vi "uTTA_SetDUT_Name.vi"(8 "error in":errorcluster, 10 "DUT Name":string, 11 "VISA Refnum in":refnum<visa-resource-name>) -> (0 "error out":errorcluster, 2 "Received":string, 3 "VISA Refnum out":refnum<visa-resource-name>)   [LabVIEW 2021]
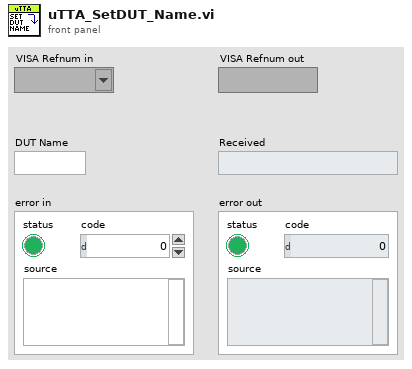
[diagram p1: front panel]
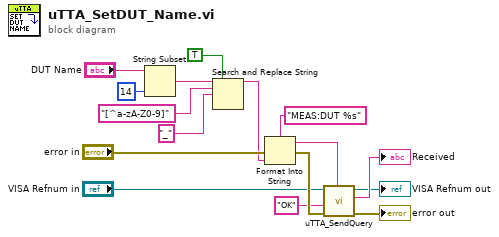
[diagram p0: block diagram]
diagram:
  n1 = String Subset(string="DUT Name", length (rest)=14 ("length (rest)")) -> (substring=w3:string)  [unwired: 1 in]
  n2 = Search and Replace String(replace all?=TRUE ("replace all? (F)"), input string=w3, search string="[^a-zA-Z0-9]", replace string="_" ("replace string (\"\")")) -> (result string=w2:string)  [unwired: 4 in, 3 out]
  n3 = Format Into String(format string="MEAS:DUT %s", error in="error in", w2) -> (resulting string=w13:string, error out=w15:errorcluster)  [unwired: 1 in]
  n4 = call "uTTA_SendQuery.vi"("Send String"=w13, "error in (no error)"=w15, "Response Qualifier(\"\")"="OK" ("Response Qualifier(\"\")"), "VISA Refnum in"="VISA Refnum in") -> ("error out"=→"error out":errorcluster, "Received"=→"Received":string, "VISA Refnum out"=→"VISA Refnum out":refnum<visa-resource-name>)  [unwired: 5 in]
